vi "ErrorHandling.Log.vi"(5 "Critical? (F)":bool, 8 "error in (no error)":errorcluster, 10 "ErrData":T2, 11 "Group":T1=enum."Gui") -> (0 "error out":errorcluster)   [LabVIEW 2014]
uses:
  CitTemplate/citTemplate.errData.ctl
  EventLog/EventLog.EventSource.ctl
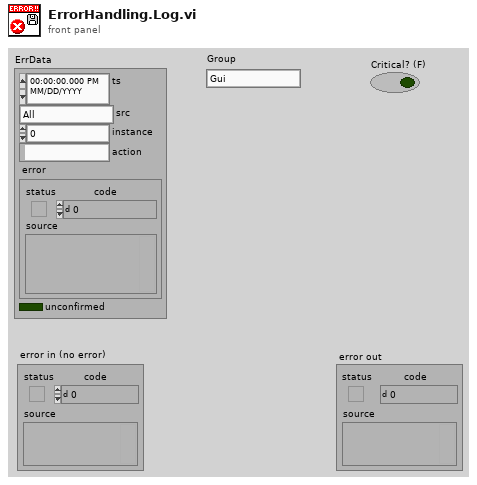
[diagram p1: front panel]
types:
  T1 = typedef "EventLog.EventSource.ctl" = enum16{"All", "Gui", "Ref", "File", "Seq", "Scan", "AO", "AI", "CI", "DIO", "M1", "M2", "Screw1", "Screw2", "Proda", "Trace"}
  T2 = typedef "citTemplate.errData.ctl" = cluster{"ts":timestamp, "src":T1, "instance":i32, "action":string, "error":errorcluster, "unconfirmed":bool}
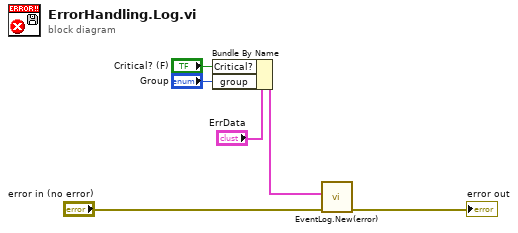
[diagram p0: block diagram]
diagram:
  n1 = Bundle By Name(cluster="ErrData", "Critical?"="Critical? (F)", "group"="Group") -> (w5:T2)
  n2 = call "EventLog.New(error).vi"("error in"="error in (no error)", "ErrData"=w5) -> ("error out"=→"error out":errorcluster)  [unwired: 9 in]
